vi "Condition Input Data.vi"(9 "Data Size":i32, 10 "Circular Buffer Size":u32, 11 "Data In":dbl[][](array[numeric])) -> (2 "Input Data Size":u32, 3 "Data In Conditioned":dbl[][](array[numeric]))   [LabVIEW 2021]
doc: "Author: Scott Hannahs <sth@magnet.fsu.edu>\nCopyright 2018 Florida State University, All rights reserved."
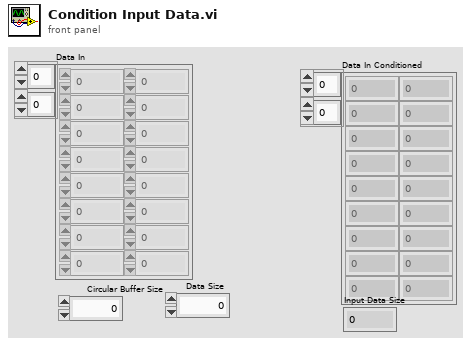
[diagram p1: front panel]
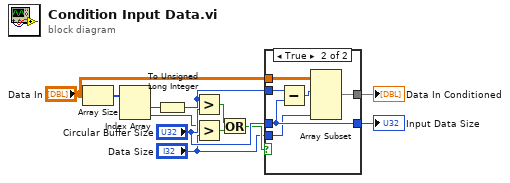
[diagram p0: block diagram]
diagram:
  n1 = Array Size(array="Data In") -> (size(s)=w12:i32[])
  n2 = Index Array(array=w12) -> (element #1=w8:i32, element #2=w4:i32)  [unwired: 2 in]
  n3 = To Unsigned Long Integer(number=w8) -> (unsigned 32bit integer=w5:u32)
  n4 = Greater?(x=w5, y="Circular Buffer Size") -> (0:w7:bool)
  n5 = Greater?(x=w4, y="Data Size") -> (0:w2:bool)
  n6 = Or(x=w7, y=w2) -> (x .or. y?=w3:bool)
  n7 = case shown="True" w3 {
    tunnel: [w14 w19] -> w11
    tunnel: "Data In" -> [w14 w20]
    tunnel: [w13 w16] -> w9
    tunnel: w5 -> [w13 w18]
    tunnel: "Circular Buffer Size" -> [_ w16]
    tunnel: "Data Size" -> [_ w15]
    frame False {
    }
    frame True {
      n8 = Subtract(x=w18, y=w16) -> (x-y=w17:u32)
      n9 = Array Subset(array=w20, index (row)=w17, length (col)=w15) -> (w19:dbl[][])  [unwired: 2 in]
    }
  }
  "Data In Conditioned" <- w11
  "Input Data Size" <- w9
